vi "Force Accuracy Test SAA.vi"(8 "error in (no error)":errorcluster, 10 "Model in":refnum<class "Model.lvclass">, 11 "Test Actuator State in":refnum<class "Test Actuator State.lvclass">) -> (0 "error out":errorcluster, 1 "Pass":bool, 2 "Model out":refnum<class "Model.lvclass">, 3 "Test Actuator State out":refnum<class "Test Actuator State.lvclass">)   [LabVIEW 2016, in "Test Actuator State.lvclass"]
uses:
  Test Actuator State.lvclass
  Model/Model/Model.lvclass
  <vilib>/Platform/TimedLoop/XDataNode/timing_clust.ctl
  <vilib>/Platform/TimedLoop/XDataNode/nitl_modes.ctl
  <vilib>/Platform/TimedLoop/XDataNode/wakeup.ctl
  Typedefs/ActuatorSetPoints.ctl
  Model/Model/Model.lvclass/Model.ctl
  <vilib>/Analysis/baseanly.llb/Mean (DBL).vi
  <vilib>/Analysis/5stat.llb/RMS (DBL).vi
  <vilib>/platform/TimedLoop/XDataNode/XDataNode.xnode
  Model/Waveforms/Waveform/Waveform.lvclass
  Typedefs/FAMT Typedefs.lvlib
  <vilib>/Analysis/NI_AALPro.lvlib
  <vilib>/Analysis/NI_AALBase.lvlib
  <vilib>/Platform/TimedLoop/XDataNode/XDNodeRunTimeDep.lvlib
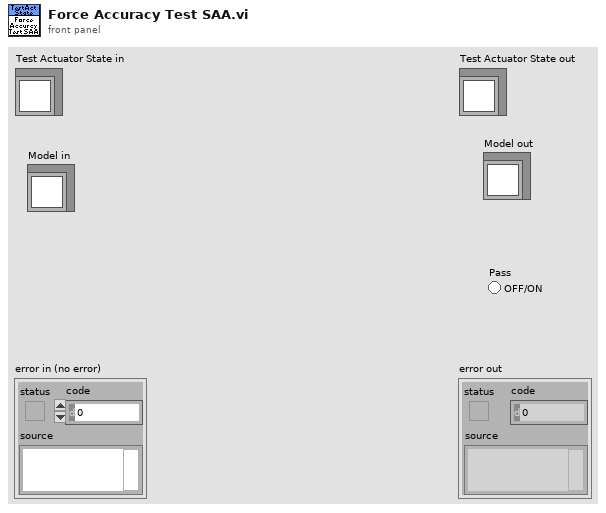
[diagram p1: front panel]
types:
  T1 = typedef "FAMT Typedefs.lvlib/ForceAccuracyTestSettings.ctl" = cluster{"Max Force Error (N)":dbl, "Max Moment (NM)":dbl, "Process Time (s)":dbl, "Sample Time (s)":dbl, "Iterations":i32, "Amplitude (N)":dbl, "Non-Repeating Error":dbl}
  T2 = typedef "XDNodeRunTimeDep.lvlib/timing_clust.ctl" = cluster{"Expected End [f-1]":u64, "Actual End [f-1]":u64, "Finished Late? [f-1]":bool, "Expected End [i-1]":u64, "Actual End [i-1]":u64, "Finished Late? [i-1]":bool, "Expected Start [i]":u64, "Actual Start [i]":u64, "Expected Start [f]":u64, "Actual Start [f]":u64, "Source Name":string, "Structure Name":string, "Period":i64, "Deadline":i64, "Offset":i64, "Start":i64, "Priority":i32, "Timeout":i32, "Mode":T3, "Wakeup Reason":T4, "Error":errorcluster, "Source Type":string, "Secondary Source Type":string, "Global End Time":u64, "Global Start Time":u64, "Frame Duration":u64, "Iteration Duration":u64, "Assigned CPU":i32, "I/O Scan Engine Mode":u32}
  T3 = typedef "XDNodeRunTimeDep.lvlib/nitl_modes.ctl" = enum32{"No Change", "Process missed periods, maintain original phase", "Discard missed periods, maintain original phase", "Process missed periods, ignore original phase", "Discard missed periods, ignore original phase"}
  T4 = typedef "XDNodeRunTimeDep.lvlib/wakeup.ctl" = enum32{"Normal", "Aborted", "Asynchronous wakeup", "Timing source error", "Timed loop error", "Timeout"}
  T5 = typedef "FAMT Typedefs.lvlib/ActuatorSetPoints.ctl" = cluster{"Axial Force":dbl, "Lateral Force":dbl, "FC1 Force":dbl, "FC2 Force":dbl}
  T6 = typedef "FAMT Typedefs.lvlib/ActuatorData.ctl" = cluster{"Timestamp":dbl, "Axial Force":dbl, "Lateral Force":dbl, "FC1 Force":dbl, "FC2 Force":dbl, "Lateral Push Pressure":dbl, "Lateral Pull Pressure":dbl, "Axial Push Pressure":dbl, "Axial Pull Pressure":dbl}
  T7 = typedef "FAMT Typedefs.lvlib/ToveyEngData.ctl" = cluster{"Timestamp":dbl, "Fx":dbl, "Fy":dbl, "Fz":dbl, "Mx":dbl, "My":dbl, "Mz":dbl}
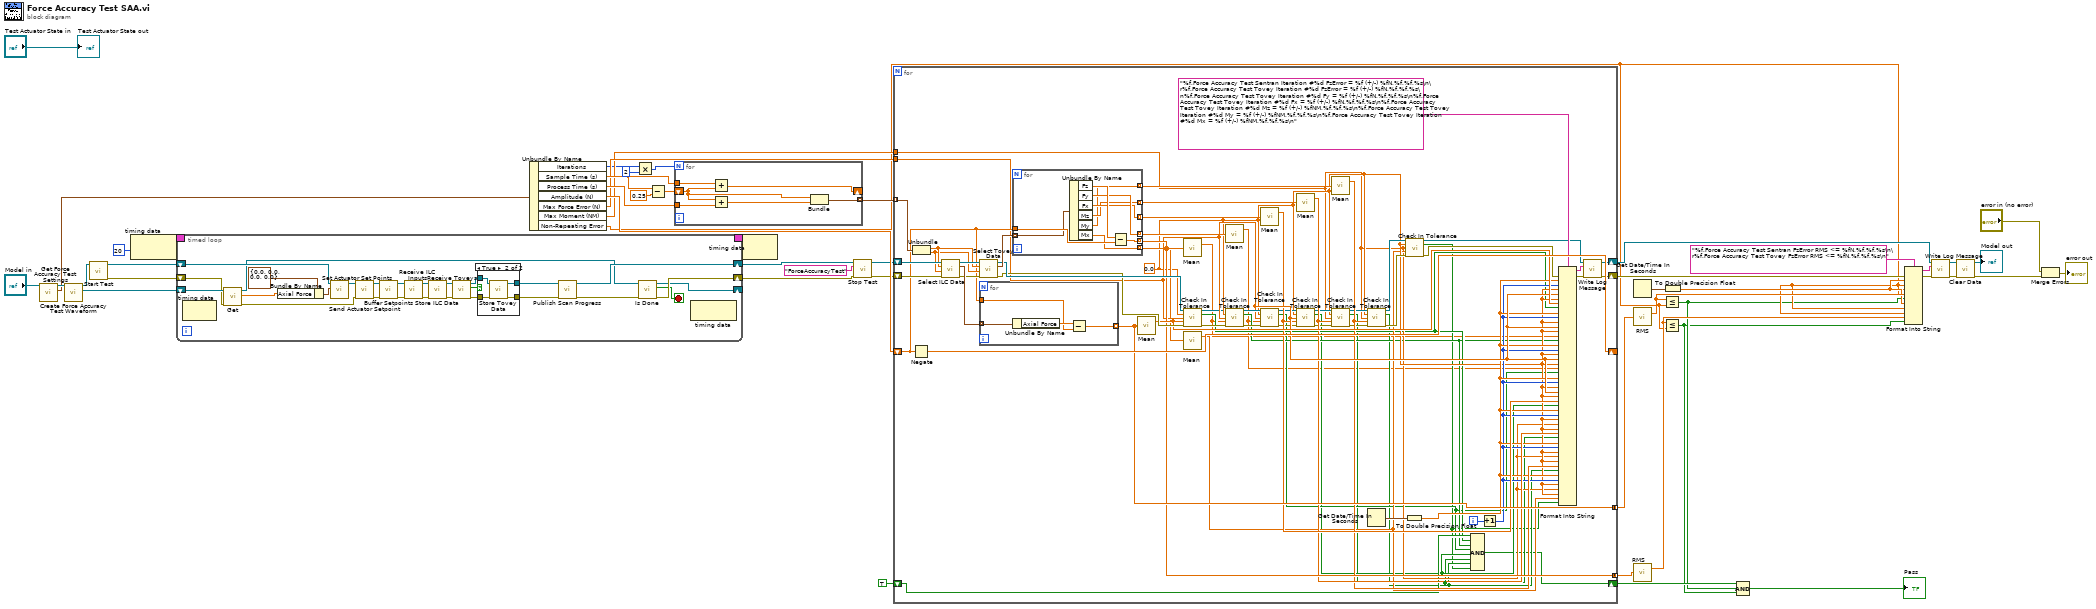
[diagram p0: block diagram]
diagram:
  n1 = call-dynamic "Get Force Accuracy Test Settings.vi"("Model in"="Model in") -> ("Force Accuracy Test Settings"=w45:T1, "Model out"=w46:refnum<class "Model.lvclass">)  [unwired: 9 in]
  n2 = call "Create Force Accuracy Test Waveform.vi"("Model in"=w46) -> ("Waveform"=w42:refnum<class "Waveform.lvclass">, "Model out"=w16:refnum<class "Model.lvclass">)  [unwired: 9 in]
  n3 = call "Start Test.vi"("Model in"=w16) -> ("error out"=w15:errorcluster, "Model out"=w14:refnum<class "Model.lvclass">)  [unwired: 9 in]
  n4 = node-c288(i64 20 ("Period")) -> (w19:T2)
  n5 = timed-loop {
    shift-right: [w75] -> w13
    shift-left: w14 -> [w67]
    shift-right: [w58] -> w11
    shift-left: w15 -> [w61]
    shift-right: [w56] -> _
    shift-left: w42 -> [w63]
    timing: w19 -> [_]
    timing-out: [_] -> w18
    stop <- w57 stop-if-true
    n6 = node-c288() -> ()  [unwired: 1 in, 1 out]
    n7 = call-dynamic "Get.vi"("error in (no error)"=w61, "Waveform in"=w63) -> ("error out"=w60:errorcluster, "Value"=w55:dbl, "Waveform out"=w62:refnum<class "Waveform.lvclass">)  [unwired: 7 in]
    n8 = Bundle By Name(cluster=T5 {"Axial Force"=0.0, "Lateral Force"=0.0, "FC1 Force"=0.0, "FC2 Force"=0.0} ("Actuator Set Points"), "Axial Force"=w55) -> (w64:T5)
    n9 = call "Set Actuator Set Points.vi"("Actuator Set Points"=w64, "Model in"=w67) -> ("Model out"=w66:refnum<class "Model.lvclass">)  [unwired: 9 in]
    n10 = call "Send Actuator Setpoint.vi"("error in (no error)"=w60, "Model in"=w66) -> ("error out"=w52:errorcluster, "Model out"=w53:refnum<class "Model.lvclass">)  [unwired: 8 in]
    n11 = call "Buffer Setpoints.vi"("error in (no error)"=w52, "Model in"=w53) -> ("error out"=w51:errorcluster, "Model out"=w54:refnum<class "Model.lvclass">)  [unwired: 8 in]
    n12 = call "Receive ILC Inputs.vi"("error in (no error)"=w51, "Model in"=w54) -> ("error out"=w76:errorcluster, "Model out"=w77:refnum<class "Model.lvclass">)  [unwired: 8 in]
    n13 = call "Store ILC Data.vi"("error in (no error)"=w76, "Model in"=w77) -> ("error out"=w73:errorcluster, "Model out"=w74:refnum<class "Model.lvclass">)  [unwired: 8 in]
    n14 = call "Receive Toveys.vi"("error in (no error)"=w73, "Model in"=w74) -> ("error out"=w71:errorcluster, "Data Received"=w70:bool, "Model out"=w72:refnum<class "Model.lvclass">)  [unwired: 7 in]
    n15 = case shown="True" w70 {
      tunnel: w72 -> [w81 w85]
      tunnel: w71 -> [w80 w84]
      tunnel: [w80 w83] -> w68
      tunnel: [w81 w82] -> w69
      frame False {
      }
      frame True {
        n16 = call "Store Tovey Data.vi"("error in (no error)"=w84, "Model in"=w85) -> ("error out"=w83:errorcluster, "Model out"=w82:refnum<class "Model.lvclass">)  [unwired: 8 in]
      }
    }
    n17 = call "Publish Scan Progress.vi"("error in (no error)"=w68, "Model in"=w69) -> ("error out"=w59:errorcluster, "Model out"=w75:refnum<class "Model.lvclass">)  [unwired: 8 in]
    n18 = call-dynamic "Is Done.vi"("error in (no error)"=w59, "Waveform in"=w62) -> ("error out"=w58:errorcluster, "Is Done"=w57:bool, "Waveform out"=w56:refnum<class "Waveform.lvclass">)  [unwired: 7 in]
    n19 = node-c288() -> ()  [unwired: 1 in, 1 out]
  }
  n20 = Unbundle By Name(w45) -> ("Iterations"=w3:i32, "Sample Time (s)"=w38:dbl, "Process Time (s)"=w39:dbl, "Amplitude (N)"=w36:dbl, "Max Force Error (N)"=w33:dbl, "Max Moment (NM)"=w32:dbl, "Non-Repeating Error"=w22:dbl)
  n21 = Multiply(x=w3, y=2) -> (x*y=w1:i32)
  n22 = Subtract(x=w38, y=0.25) -> (x-y=w40:dbl)
  n23 = for {
    N: w1 -> [_]
    shift-right: [w89] -> _
    shift-left: w40 -> [w87]
    tunnel: w39 -> [w91]
    tunnel: w38 -> [w90]
    tunnel: [w86] -> w37 mode=indexing
    n24 = Add(x=w90, y=w87) -> (x+y=w89:dbl)
    n25 = Add(x=w87, y=w91) -> (x+y=w88:dbl)
    n26 = Bundle(w87, w88) -> (w86:cluster{dbl, dbl})  [unwired: 1 in]
  }
  n27 = node-c288(w18) -> ()  [unwired: 1 out]
  n28 = call "Stop Test.vi"("error in (no error)"=w11, "Test"="ForceAccuracyTest", "Model in"=w13) -> ("error out"=w10:errorcluster, "Model out"=w12:refnum<class "Model.lvclass">)  [unwired: 7 in]
  n29 = for {
    tunnel: w37 -> [w153] mode=indexing
    shift-right: [w134] -> w25
    shift-left: w12 -> [w152]
    shift-right: [w150] -> _
    shift-left: w36 -> [w132]
    tunnel: [w140] -> w35 mode=concatenating
    shift-right: [w135] -> w28
    shift-left: w10 -> [w149]
    tunnel: [w131] -> w34 mode=concatenating
    tunnel: w33 -> [w126]
    tunnel: w32 -> [w105]
    shift-right: [w94] -> w7
    shift-left: TRUE -> [w102]
    i -> [w141]
    w107 = 0.0
    n30 = Negate(x=w132) -> (-x=w150:dbl)
    n31 = Unbundle(w153) -> (w147:dbl, w146:dbl)
    n32 = call "Select ILC Data.vi"("error in (no error)"=w149, "End Time"=w146, "Start Time"=w147, "Model in"=w152) -> ("error out"=w145:errorcluster, "Data"=w151:T6[], "Model out"=w148:refnum<class "Model.lvclass">)  [unwired: 4 in, 1 out]
    n33 = call "Select Tovey Data.vi"("error in (no error)"=w145, "End Time"=w146, "Start Time"=w147, "Model in"=w148) -> ("error out"=w138:errorcluster, "Data"=w144:T7[], "Model out"=w139:refnum<class "Model.lvclass">)  [unwired: 4 in, 1 out]
    n34 = for {
      tunnel: w151 -> [w166] mode=indexing
      tunnel: w132 -> [w163]
      tunnel: [w164] -> w140 mode=indexing
      n35 = Unbundle By Name(w166) -> ("Axial Force"=w165:dbl)
      n36 = Subtract(x=w165, y=w163) -> (x-y=w164:dbl)
    }
    n37 = for {
      tunnel: w132 -> [w159]
      tunnel: [w161] -> w131 mode=indexing
      tunnel: [w160] -> w130 mode=indexing
      tunnel: [w158] -> w127 mode=indexing
      tunnel: [w157] -> w122 mode=indexing
      tunnel: [w156] -> w118 mode=indexing
      tunnel: [w155] -> w112 mode=indexing
      tunnel: w144 -> [w154] mode=indexing
      n38 = Unbundle By Name(w154) -> ("Fz"=w162:dbl, "Fy"=w160:dbl, "Fx"=w158:dbl, "Mz"=w157:dbl, "My"=w156:dbl, "Mx"=w155:dbl)
      n39 = Subtract(x=w162, y=w159) -> (x-y=w161:dbl)
    }
    n40 = call-poly <vilib>:"Mean.vi"("X"=w140) -> ("mean"=w137:dbl)  [unwired: 1 out]
    n41 = call-poly <vilib>:"Mean.vi"("X"=w131) -> ("mean"=w92:dbl)  [unwired: 1 out]
    n42 = call "Check In Tolerance.vi"("Model in"=w139, "Expected"=w107, "Tolerance"=w126, "Actual"=w137, "error in (no error)"=w138) -> ("Model out"=w104:refnum<class "Model.lvclass">, "Pass"=w101:bool, "error out"=w103:errorcluster)  [unwired: 8 in]
    n43 = call-poly <vilib>:"Mean.vi"("X"=w112) -> ("mean"=w106:dbl)  [unwired: 1 out]
    n44 = call-poly <vilib>:"Mean.vi"("X"=w130) -> ("mean"=w93:dbl)  [unwired: 1 out]
    n45 = call "Check In Tolerance.vi"("Model in"=w104, "Expected"=w107, "Tolerance"=w126, "Actual"=w92, "error in (no error)"=w103) -> ("Model out"=w129:refnum<class "Model.lvclass">, "Pass"=w100:bool, "error out"=w128:errorcluster)  [unwired: 8 in]
    n46 = call-poly <vilib>:"Mean.vi"("X"=w127) -> ("mean"=w125:dbl)  [unwired: 1 out]
    n47 = call "Check In Tolerance.vi"("Model in"=w129, "Expected"=w107, "Tolerance"=w126, "Actual"=w93, "error in (no error)"=w128) -> ("Model out"=w124:refnum<class "Model.lvclass">, "Pass"=w99:bool, "error out"=w123:errorcluster)  [unwired: 8 in]
    n48 = call-poly <vilib>:"Mean.vi"("X"=w122) -> ("mean"=w121:dbl)  [unwired: 1 out]
    n49 = call "Check In Tolerance.vi"("Model in"=w124, "Expected"=w107, "Tolerance"=w126, "Actual"=w125, "error in (no error)"=w123) -> ("Model out"=w120:refnum<class "Model.lvclass">, "Pass"=w98:bool, "error out"=w119:errorcluster)  [unwired: 8 in]
    n50 = call-poly <vilib>:"Mean.vi"("X"=w118) -> ("mean"=w117:dbl)  [unwired: 1 out]
    n51 = call "Check In Tolerance.vi"("Model in"=w120, "Expected"=w107, "Tolerance"=w105, "Actual"=w121, "error in (no error)"=w119) -> ("Model out"=w116:refnum<class "Model.lvclass">, "Pass"=w97:bool, "error out"=w115:errorcluster)  [unwired: 8 in]
    n52 = call "Check In Tolerance.vi"("Model in"=w116, "Expected"=w107, "Tolerance"=w105, "Actual"=w117, "error in (no error)"=w115) -> ("Model out"=w111:refnum<class "Model.lvclass">, "Pass"=w96:bool, "error out"=w109:errorcluster)  [unwired: 8 in]
    n53 = Get Date/Time In Seconds() -> (seconds since 1Jan1904=w142:timestamp)
    n54 = To Double Precision Float(number=w142) -> (double precision float=w114:dbl)
    n55 = call "Check In Tolerance.vi"("Model in"=w111, "Expected"=w107, "Tolerance"=w105, "Actual"=w106, "error in (no error)"=w109) -> ("Model out"=w110:refnum<class "Model.lvclass">, "Pass"=w95:bool, "error out"=w108:errorcluster)  [unwired: 8 in]
    n56 = Compound Arithmetic op=AND(w102, w101, w100, w99, w98, w97, w96, w95) -> (w94:bool)
    n57 = Increment(x=w141) -> (x+1=w113:i32)
    n58 = Format Into String(format string="%f,Force Accuracy Test Sentran Iteration #%d FzError = %f (+/-) %fN,%f,%f,%s\n\r%f,Force Accuracy Test Tovey Iteration #%d FzError = %f (+/-) %fN,%f,%f,%s\n%f,Force Accuracy Test Tovey Iteration #%d Fy = %f (+/-) %fN,%f,%f,%s\n%f,Force Accuracy Test Tovey Iteration #%d Fx = %f (+/-) %fN,%f,%f,%s\n%f,Force Accuracy Test Tovey Iteration #%d Mz = %f (+/-) %fNM,%f,%f,%s\n%f,Force Accuracy Test Tovey Iteration #%d My = %f (+/-) %fNM,%f,%f,%s\n%f,Force Accuracy Test Tovey Iteration #%d Mx = %f (+/-) %fNM,%f,%f,%s\n", error in=w108, w114, w113, w107, w126, w107, w137, w101, w114, w113, w107, w126, w107, w92, w100, w114, w113, w107, w126, w107, w93, w99, w114, w113, w107, w126, w107, w125, w98, w114, w113, w107, w105, w107, w121, w97, w114, w113, w107, w105, w107, w117, w96, w114, w113, w107, w105, w107, w106, w95) -> (resulting string=w133:string, error out=w136:errorcluster)  [unwired: 1 in]
    n59 = call "Write Log Message.vi"("error in (no error)"=w136, "Message"=w133, "Model in"=w110) -> ("error out"=w135:errorcluster, "Model out"=w134:refnum<class "Model.lvclass">)  [unwired: 7 in]
  }
  n60 = Get Date/Time In Seconds() -> (seconds since 1Jan1904=w30:timestamp)
  n61 = call-poly <vilib>:"RMS.vi"("X"=w35) -> ("rms value"=w29:dbl)  [unwired: 1 out]
  n62 = call-poly <vilib>:"RMS.vi"("X"=w34) -> ("rms value"=w24:dbl)  [unwired: 1 out]
  n63 = Less Or Equal?(x=w29, y=w22) -> (x <= y?=w6:bool)
  n64 = Less Or Equal?(x=w24, y=w22) -> (x <= y?=w5:bool)
  n65 = To Double Precision Float(number=w30) -> (double precision float=w23:dbl)
  n66 = Compound Arithmetic op=AND(w7, w6, w5) -> (→"Pass":bool)
  n67 = Format Into String(format string="%f,Force Accuracy Test Sentran FzError RMS <= %fN,%f,%f,%s\n\r%f,Force Accuracy Test Tovey FzError RMS <= %fN,%f,%f,%s\n", error in=w28, w23, w22, w22, w29, w6, w23, w22, w22, w24, w5) -> (resulting string=w26:string, error out=w27:errorcluster)  [unwired: 1 in]
  n68 = call "Write Log Message.vi"("error in (no error)"=w27, "Message"=w26, "Model in"=w25) -> ("error out"=w21:errorcluster, "Model out"=w20:refnum<class "Model.lvclass">)  [unwired: 7 in]
  n69 = call "Clear Data.vi"("error in (no error)"=w21, "Model in"=w20) -> ("error out"=w44:errorcluster, "Model out"=→"Model out":refnum<class "Model.lvclass">)  [unwired: 8 in]
  n70 = Merge Errors("error in (no error)", w44) -> (→"error out":errorcluster)
  "Test Actuator State out" <- "Test Actuator State in"
